vi "Get Sun App Long.vi"(9 "Sun Eq of Ctr":dbl, 10 "Julian Century":dbl, 11 "Geometric Mean Longitude":dbl) -> (2 "Sun App Long (deg)":dbl, 3 "Sun True Longitude":dbl)   [LabVIEW 2014, in "Solar Calculations.lvlib"]
uses:
  Solar Calculations.lvlib
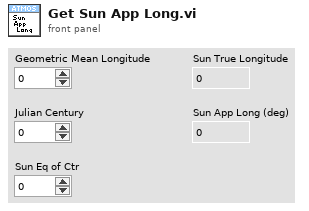
[diagram p1: front panel]
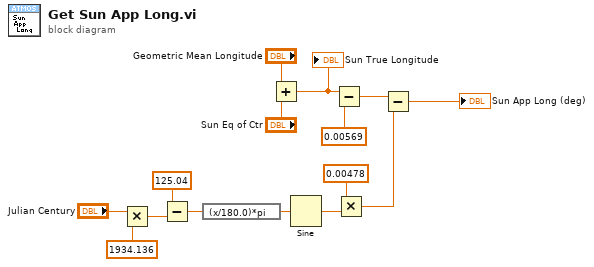
[diagram p0: block diagram]
diagram:
  n1 = Multiply(x="Julian Century", y=1934.136) -> (x*y=w8:dbl)
  n2 = Subtract(x=125.04, y=w8) -> (x-y=w10:dbl)
  n3 = expression code="(x/180.0)*pi" ("degrees to radians")(w10) -> (w11:dbl)
  n4 = Add(x="Geometric Mean Longitude", y="Sun Eq of Ctr") -> (x+y=w3:dbl)
  "Sun True Longitude" <- w3
  n5 = Sine(x=w11) -> (sin(x)=w12:dbl)
  n6 = Subtract(x=w3, y=0.00569) -> (x-y=w5:dbl)
  n7 = Multiply(x=0.00478, y=w12) -> (x*y=w14:dbl)
  n8 = Subtract(x=w5, y=w14) -> (x-y=→"Sun App Long (deg)":dbl)
